vi "Enqueue Message.vi"(8 "Error In":errorcluster, 10 "Message":T1, 11 "Process In":refnum<class "Process.lvclass">) -> (0 "Error Out":errorcluster, 3 "Process Out":refnum<class "Process.lvclass">)   [LabVIEW 2021, in "Process.lvclass"]
uses:
  Process.lvclass
  Central Message Handler/Public/Controls/Message.ctl
  Accessors/Central Message Handler Queue/Get Central Message Handler Queue.vi
  Central Message Handler/Central Message Handler.lvclass
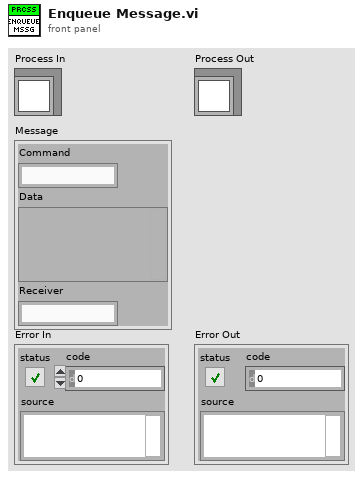
[diagram p1: front panel]
types:
  T1 = typedef "Central Message Handler.lvclass/Message.ctl" = cluster{"Command":string, "Data":variant, "Receiver":string}
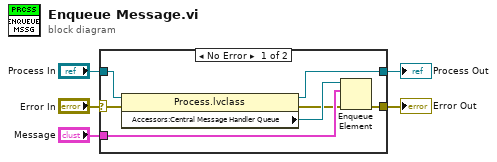
[diagram p0: block diagram]
diagram:
  n1 = case shown="No Error" "Error In" {
    selector: "Error In" -> [w6 w13]
    tunnel: [w12 w13] -> w5
    tunnel: [w11 w14] -> w4
    tunnel: "Message" -> [w10 _]
    tunnel: "Process In" -> [w7 w14]
    frame No Error {
      n2 = property class="Process.lvclass"(reference=w7, error in=w6) -> (reference out=w11:refnum<class "Process.lvclass">, error out=w8:errorcluster, "Accessors:Central Message Handler Queue"=w9:refnum<queue>)
      n3 = Enqueue Element(queue=w9, element=w10, error in (no error)=w8) -> (error out=w12:errorcluster)  [unwired: 1 in, 2 out]
    }
    frame Error {
    }
  }
  "Error Out" <- w5
  "Process Out" <- w4
